vi "reset FPGA DMA.vi"(2 "error in":errorcluster, 3 "FPGA VI Reference In":T1) -> (0 "error out":errorcluster, 1 "FPGA VI Reference Out":T1)   [LabVIEW 2014]
uses:
  <vilib>/rvi/interface/nirviReadWriteControl/nirviReadWriteControl.xnode
  openfpgaref.8.6.ctl
  <vilib>/rvi/interface/nirviMethod/nirviMethod.xnode
  <vilib>/rvi/errors/niLvFpgaMergeErrorWithErrorCode.vi
  <vilib>/FPGAPlugInAG/PCIe-7852R/niLvFpga_StopFifo_PCIe-7852R.vi
  <vilib>/FPGAPlugInAG/PCIe-7852R/niLvFpga_StartFifo_PCIe-7852R.vi
  FPGA Bitfiles/UHR-FleezersInst_FPGATarget_UHR-FleezersCont_IqK95Pvv9lYv5.3.lvbitx
  NiFpgaLv.dll
  <vilib>/Utility/error.llb/Error Cluster From Error Code.vi
  <vilib>/rvi/errors/niLvFpgaAdjustHostInterfaceError.vi
panel:
  out "Overflow (data lost)":bool
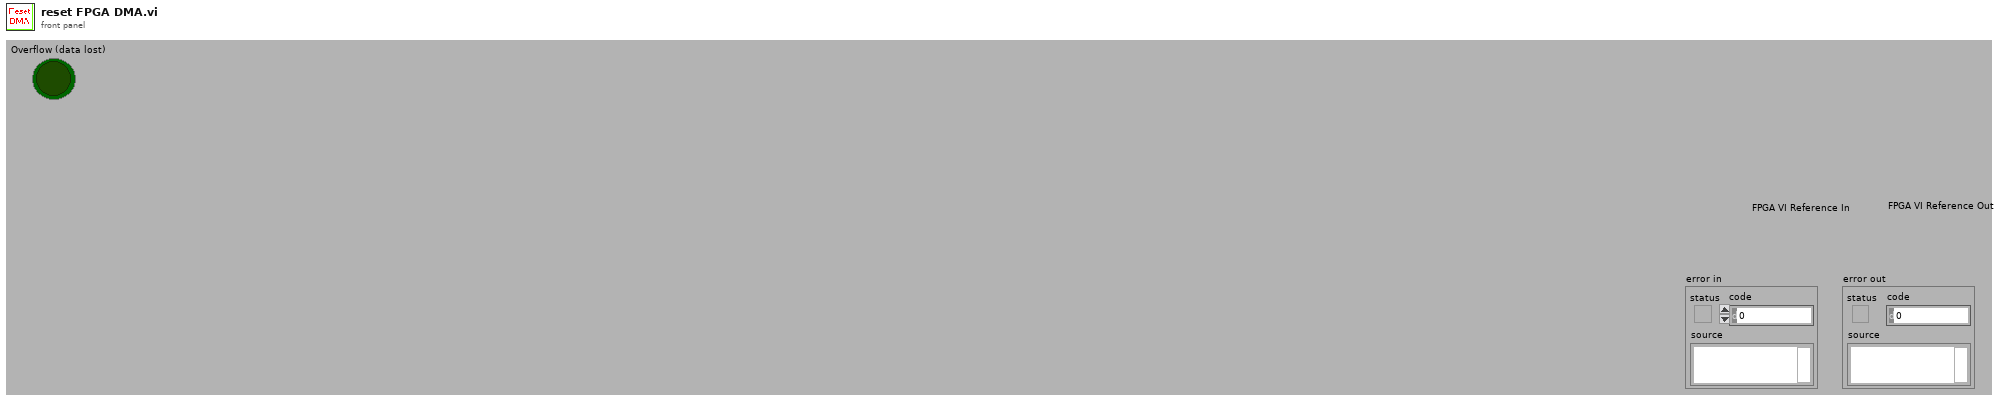
[diagram p1: front panel]
types:
  T1 = typedef "openfpgaref.8.6.ctl" = refnum<k20>
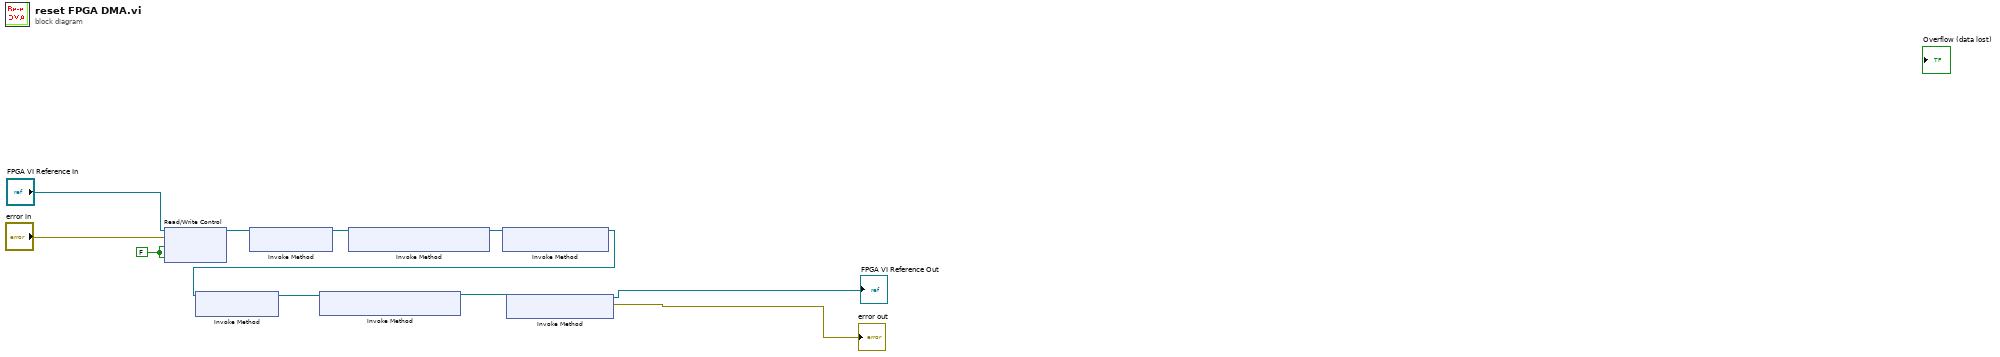
[diagram p0: block diagram]
diagram:
  w11 = FALSE ("AI to FIFO")
  n1 = xnode "Read/Write Control"("FPGA VI Reference In"="FPGA VI Reference In", "error in"="error in", "AI to FIFO"=w11, "APD to FIFO"=w11) -> ("FPGA VI Reference Out"=w5:T1)  [unwired: 1 out]
  n2 = xnode "Invoke Method"("FPGA VI Reference In"=w5) -> ("FPGA VI Reference Out"=w10:T1)  [unwired: 1 in, 1 out]
  n3 = xnode "Invoke Method"("FPGA VI Reference In"=w10) -> ("FPGA VI Reference Out"=w9:T1)  [unwired: 1 in, 1 out]
  n4 = xnode "Invoke Method"("FPGA VI Reference In"=w9) -> ("FPGA VI Reference Out"=w8:T1)  [unwired: 1 in, 1 out]
  n5 = xnode "Invoke Method"("FPGA VI Reference In"=w8) -> ("FPGA VI Reference Out"=w4:T1)  [unwired: 1 in, 1 out]
  n6 = xnode "Invoke Method"("FPGA VI Reference In"=w4) -> ("FPGA VI Reference Out"=w3:T1)  [unwired: 1 in, 1 out]
  n7 = xnode "Invoke Method"("FPGA VI Reference In"=w3) -> ("FPGA VI Reference Out"=→"FPGA VI Reference Out":T1, "error out"=→"error out":errorcluster)  [unwired: 1 in]
